vi "Update Bus B Data.vi"(5 "Component ID":u8, 7 "FPGA Interface":refnum<class "FPGA Interface.lvclass">, 8 "error in (no error)":errorcluster, 11 "Bus Monitor in":refnum<class "Bus Monitor.lvclass">) -> (0 "error out":errorcluster, 3 "Bus Monitor out":refnum<class "Bus Monitor.lvclass">)   [LabVIEW 2020, in "BCI-1553 API.lvlib" / "Bus Monitor.lvclass"]
doc: "Updates all the data values in filter parameters for Bus B. The data is stored in memory in a haphazardous manner, so we need to know a lot of information about the filter definition to retrieve the values correctly. It's also not quite ideal to have to make a public accessor for writing parameters. That could hurt later, but it works well to this means."
uses:
  Bus Monitor.lvclass
  Dependencies/FPGA Interface/FPGA Interface.lvclass
  Bus Monitor.lvclass/Bus Monitor.ctl
  Dependencies/Registry/Registry.lvclass/Registry.ctl
  Filters/Filter/Filter.lvclass
  Dependencies/Registry/Add Entry.vi
  Dependencies/Registry/Registry.lvclass
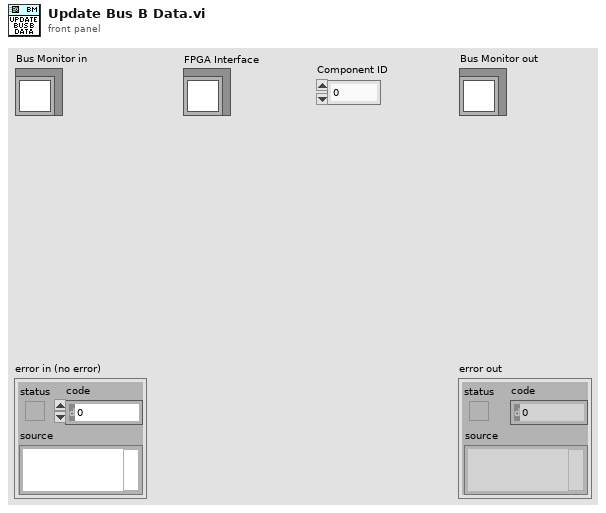
[diagram p1: front panel]
types:
  T1 = typedef "BCI-1553 API.lvlib/Command Type.ctl" = enum16{"Transmit", "Receive"}
  T2 = typedef "BCI-1553 API.lvlib/Parameter Table Data.ctl" = cluster{"Parameter Name":string, "Base Word":u16, "Address":u16, "Value":u64, "Mask":u16[], "Scaling Info":T3}
  T3 = typedef "BCI-1553 API.lvlib/Scaling Information.ctl" = cluster{"Bit Offset":i32, "Bit Count":i32, "LSB Resolution":dbl, "2's Complement":bool, "Big Endian":bool, "Sign Bit":bool}
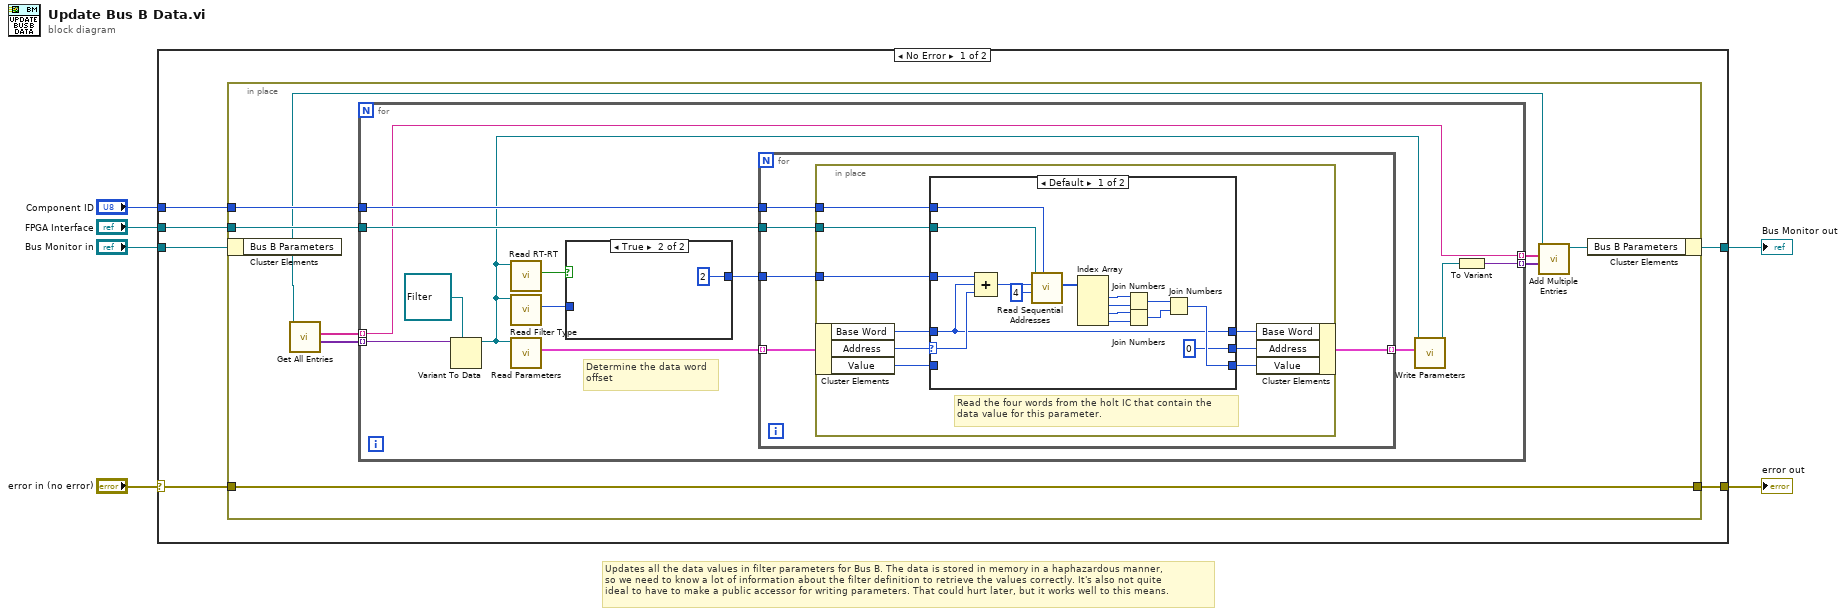
[diagram p0: block diagram]
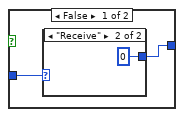
[diagram p2: hidden frame]
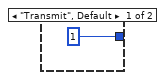
[diagram p3: hidden frame]
diagram:
  # "Updates all the data values in filter parameters for Bus B. The data is stored in memory in a haphazardous manner,\nso we need to know a lot of information about the filter definition to retrieve the values correctly. It's also not quite\nideal to have to make a public accessor for writing parameters. That could hurt later, but it works well to this means."
  n1 = case shown="No Error" "error in (no error)" {
    selector: "error in (no error)" -> [w10 w74]
    tunnel: [w9 w74] -> w1
    tunnel: [w11 w73] -> w2
    tunnel: "Bus Monitor in" -> [w12 w73]
    tunnel: "Component ID" -> [w8 _]
    tunnel: "FPGA Interface" -> [w7 _]
    frame No Error {
      n2 = in-place {
        in-place-border: w10 -> [w21]
        in-place-border: [w21] -> w9
        in-place-border: w8 -> [w18]
        in-place-border: w7 -> [w17]
        n3 = in-place-cluster #1(w12) -> ("Bus B Parameters"=w14:refnum<class "Registry.lvclass">)
        n4 = call "Get All Entries.vi"("Registry in"=w14) -> ("Values"=w20:variant[], "Keys"=w19:string[])  [unwired: 8 in, 1 out]
        n5 = for {
          tunnel: w20 -> [w34] mode=indexing
          tunnel: w19 -> [w26] mode=indexing
          tunnel: w18 -> [w32]
          tunnel: w17 -> [w31]
          tunnel: [w26] -> w16 mode=indexing
          tunnel: [w22] -> w15 mode=indexing
          # "Determine the data word\noffset"
          n6 = Variant To Data(type=refnum<class "Filter.lvclass"> refnum ("SLSC 1553 API.lvlib:Filter.lvclass"), Variant=w34) -> (data=w23:refnum<class "Filter.lvclass">)  [unwired: 1 in, 1 out]
          n7 = call-dynamic "Read RT-RT.vi"("Filter in"=w23) -> ("RT-RT"=w29:bool)  [unwired: 8 in, 2 out]
          n8 = call-dynamic "Read Filter Type.vi"("Filter in"=w23) -> ("Command Type"=w28:T1)  [unwired: 8 in, 2 out]
          n9 = call-dynamic "Read Parameters.vi"("Filter in"=w23) -> ("Parameters"=w30:T2[])  [unwired: 8 in, 2 out]
          n10 = case shown="True" w29 {
            tunnel: w28 -> [w36 _]
            tunnel: [w35 u16 2] -> w27
            frame False {
              n11 = case shown="\"Receive\"" w36 {
                tunnel: [u16 1 u16 0] -> w35
                frame "Transmit", Default {
                }
                frame "Receive" {
                }
              }
            }
            frame True {
            }
          }
          n12 = for {
            tunnel: w32 -> [w43]
            tunnel: w31 -> [w42]
            tunnel: w30 -> [w44] mode=indexing
            tunnel: w27 -> [w41]
            tunnel: [w40] -> w25 mode=indexing
            n13 = in-place {
              in-place-border: w43 -> [w50]
              in-place-border: w42 -> [w49]
              in-place-border: w41 -> [w48]
              # "Read the four words from the holt IC that contain the\ndata value for this parameter."
              n14 = in-place-cluster #2(w44) -> ("Base Word"=w47:u16, "Address"=w53:u16, "Value"=w51:u64)
              n15 = case shown="Default" w53 {
                selector: w53 -> [w56 w70]
                tunnel: [w57 w72] -> w52
                tunnel: w51 -> [_ w72]
                tunnel: w50 -> [w59 _]
                tunnel: w49 -> [w58 _]
                tunnel: w48 -> [w69 _]
                tunnel: w47 -> [w55 w71]
                tunnel: [u16 0 ("Address") w70] -> w46
                tunnel: [w55 w71] -> w45
                frame Default {
                  n16 = Compound Arithmetic op=ADD(w69, w55, w56) -> (w60:u16)
                  n17 = call-dynamic "Read Sequential Addresses.vi"("Target IC (1-8)"=w59, "Addresses to Read"=u16 4, "Starting Address"=w60, "FPGA Interface in"=w58) -> ("Data"=w67:u16[])  [unwired: 6 in, 1 out]
                  n18 = Index Array(array=w67) -> (element #1=w63:u16, element #2=w64:u16, element #3=w62:u16, element #4=w61:u16)  [unwired: 4 in]
                  n19 = Join Numbers(hi=w63, lo=w64) -> ((hi.lo)=w65:u32)
                  n20 = Join Numbers(hi=w62, lo=w61) -> ((hi.lo)=w66:u32)
                  n21 = Join Numbers(hi=w65, lo=w66) -> ((hi.lo)=w57:u64)
                }
                frame 0 {
                  # "Address word is zero. Do nothing."
                }
              }
              n22 = in-place-cluster #2("Base Word"=w45, "Address"=w46, "Value"=w52) -> (w40:T2)
            }
          }
          n23 = call-dynamic "Write Parameters.vi"("Parameters"=w25, "Filter in"=w23) -> ("Filter out"=w24:refnum<class "Filter.lvclass">)  [unwired: 8 in, 1 out]
          n24 = To Variant(anything=w24) -> (Variant=w22:variant)
        }
        n25 = call "Add Multiple Entries.vi"("Values"=w15, "Keys"=w16, "Registry in"=w14) -> ("Registry out"=w13:refnum<class "Registry.lvclass">)  [unwired: 6 in, 2 out]
        n26 = in-place-cluster #1("Bus B Parameters"=w13) -> (w11:refnum<class "Bus Monitor.lvclass">)
      }
    }
    frame Error {
    }
  }
  "error out" <- w1
  "Bus Monitor out" <- w2
